vi "LDF Get Frame Quantity.vi"(11 "LDFHandle":u64) -> (3 "function return":i32)   [LabVIEW 2010, in "ldf_parser.lvlib"]
doc: "int WINAPI LDF_GetFrameQuantity(long long LDFHandle);"
uses:
  ldf_parser.lvlib
  USB2XXX/trunk/USB2XXX/USB2XXX/vs2019/Release/USB2XXX.dll
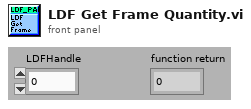
[diagram p1: front panel]
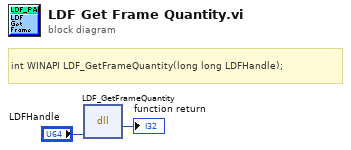
[diagram p0: block diagram]
diagram:
  # "int WINAPI LDF_GetFrameQuantity(long long LDFHandle);"
  n1 = dll-call lib="E:/Projects/USB2XXX/trunk/USB2XXX/USB2XXX/vs2019/Release/USB2XXX.*" fn="LDF_GetFrameQuantity"("LDFHandle"="LDFHandle") -> (→"function return":i32)  [unwired: 4 in, 2 out]
